vi "setPositionServo.vi"(0 "speed":u8 max=63 step=1, 1 "servo position":u16(knob)=260 max=2500 step=1 scale=0.0..2500.0, 2 "channel":u8 max=15 step=1) -> ()   [LabVIEW 2011]
uses:
  GlobalSerial.vi
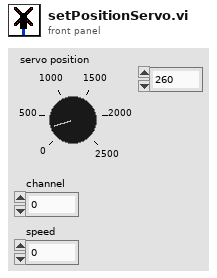
[diagram p1: front panel]
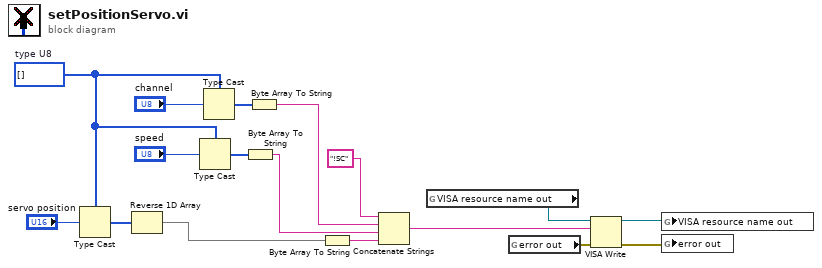
[diagram p0: block diagram]
diagram:
  w10 = u8[] []  # type U8
  n1 = Type Cast(type=w10, x="servo position") -> (*(type *) &x=w14:u8[])
  n2 = Reverse 1D Array(array=w14) -> (reversed array=w6:u8[])
  n3 = Type Cast(type=w10, x="speed") -> (*(type *) &x=w9:u8[])
  n4 = Type Cast(type=w10, x="channel") -> (*(type *) &x=w12:u8[])
  n5 = Byte Array To String(unsigned byte array=w9) -> (string=w8:string)
  n6 = Byte Array To String(unsigned byte array=w12) -> (string=w13:string)
  n7 = Byte Array To String(unsigned byte array=w6) -> (string=w15:string)
  n8 = Concatenate Strings("!SC" ("string"), w13, w8, w15) -> (w5:string)
  n9 = global read "GlobalSerial.vi" "VISA resource name out"() -> (w2:refnum<visa-resource-name>)
  n10 = global read "GlobalSerial.vi" "error out"() -> (w4:errorcluster)
  n11 = VISA Write(VISA resource name=w2, write buffer=w5, error in (no error)=w4) -> (VISA resource name out=w1:refnum<visa-resource-name>, error out=w3:errorcluster)  [unwired: 1 out]
  n12 = global write "GlobalSerial.vi" "VISA resource name out"(w1) -> ()
  n13 = global write "GlobalSerial.vi" "error out"(w3) -> ()
